vi "GUID Lookup.vi"() -> ()   [LabVIEW 2015, in "Diagnostics Addon Shared.lvlib"]
doc: "Use this Global VI to access the GUIDs assigned to the page resources of the Custom Device."
uses:
  Diagnostics Addon Shared.lvlib
panel:
  in  "Data by Identifier Page":string="Data by Identifiers"
  in  "Protected Signal GUID":string="edc2e041-ff43-4610-a968-1d89a067df1d"
  in  "Signal GUID":string="813ed40a-6aa8-4ff9-92f7-887fb6dec76c"
  in  "DB Alias":string="Diagnostics_Addon_Temp_DB"
  in  "CD Version":string="4.0.0"
  in  "Bitfile 986x":string="Bitfile 986x"
  in  "RT Bitfile Location":path=path "c:/ni-rt/NIVeriStand/XNET"
  in  "RIO Device 986x":string="RIO Device 986x"
  in  "Enable 986x":string="Enable 986x"
  in  "PID Outputs Page":string="Outputs"
  in  "PID Outputs GUID":string="edf3a6ba-361e-4d29-8f85-616268b5a338"
  in  "CommandChannels":string[](array[string])=["Command", "MetaData1", "MetaData2", "MetaData3", "MetaData4"]
  in  "ResponseQKey":string="Response"
  in  "XNETEngineSuffix":string="_XNETEngine"
  in  "CmdEngineSuffix":string="_BufferedCmds"
  in  "LookupTableConvertPrefix":string="Convert"
  in  "LookupTableSignalsPrefix":string="SignalDefs"
  in  "Diagnostics_Disable":string="1dbbfb91-19dd-4678-8b23-0ef3a754a66d"
  in  "DIDs Page":string="DIDs"
  in  "DID GUID":string="465d9377-cb59-4ae9-97ed-bc842761823f"
  in  "DIDs GUID":string="ae6faf55-1aff-4d2a-b6e8-d238aa342751"
  in  "DTC_Signals to Create":i32=10
  in  "DTC_Signal Prefix":string="DTC_"
  in  "DTC_Signal Suffix":string[](array[string])=["_Timestamp", "_Value", "_Status", "_Failure"]
  in  "DTC GUID":string="7ba6be2c-4857-4b46-8446-f293283a3924"
  in  "Diagnostic Command Success":string="Diagnostic Command Success"
  in  "DTC Descriptor":string="DTC Descriptor"
  in  "DPID Parameters":string="DPID Parameters"
  in  "DPIDs Page":string="DPIDs"
  in  "DPID GUID":string="be84dd52-6fa5-4162-93da-bfddf126599b"
  in  "DPIDs GUID":string="186cc3e9-a602-40ff-b933-3b68f6fbfaf8"
  in  "CAN Parameters":string="CAN Parameters"
  in  "DTCs_# of DTCs":string="# of DTCs"
  in  "DTCs_Masks":string="DTC Masks"
  in  "DIDPID Signal Parameters":string="Start Bit"
  in  "DIDPID_ID":string="DIDPID ID"
  in  "PID Inputs Page":string="Inputs"
  in  "PID Inputs GUID":string="3a9eaf02-736d-4e36-bf88-b98c7e9eb737"
  in  "Commands Page":string="Commands"
  in  "Services Page":string="Services"
  in  "Status Page":string="Status"
  in  "DTCs Page":string="DTCs"
  in  "PIDs Page":string="PIDs"
  in  "PID GUID":string="6b934904-49a9-4798-a421-a2da3be45ca1"
  in  "Commands GUID":string="14802196-9eef-416a-8ce6-e6467da1d504"
  in  "Status GUID":string="f7446a49-c995-4f37-8203-8e2b918d40c6"
  in  "Services GUID":string="846f9e44-937b-4fbd-9977-3745ffc89e9c"
  in  "PIDs GUID":string="1514cba4-fa1e-47dd-8223-616adb9fb21d"
  in  "DTCs GUID":string="631db7b8-0b52-4af9-934d-144228c2dbd8"
  in  "Diagnostics_Enable":string="4e42e445-e1c9-40fb-b144-894b15ca645a"
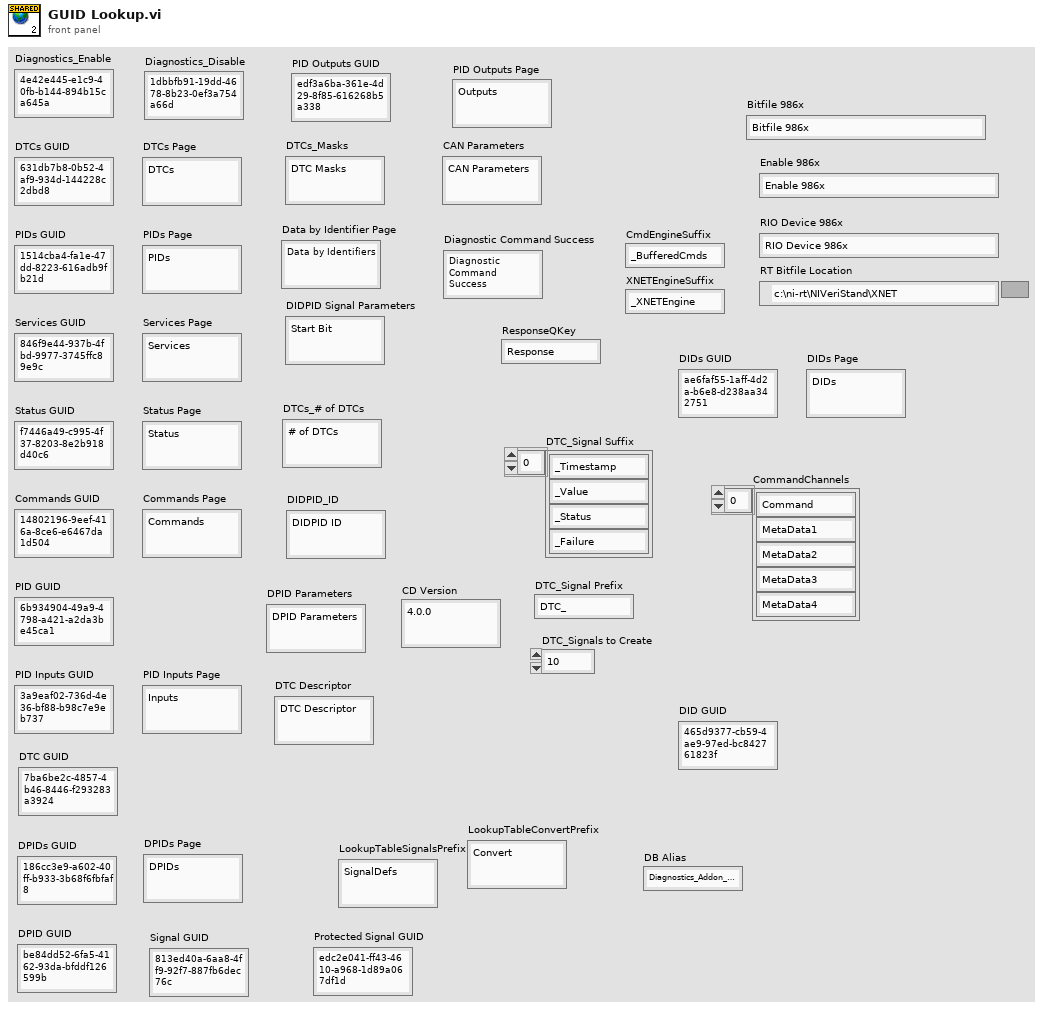
[diagram p1: front panel]
diagram:
